vi "Material-Application-Dir-Metrics.vi"(11 "error in":errorcluster) -> (4 "Metrics Log Directory":path, 15 "error out":errorcluster)   [LabVIEW 2013]
uses:
  Material-Application-Dir-User.vi
panel:
  # "Inputs"
  # "Outputs"
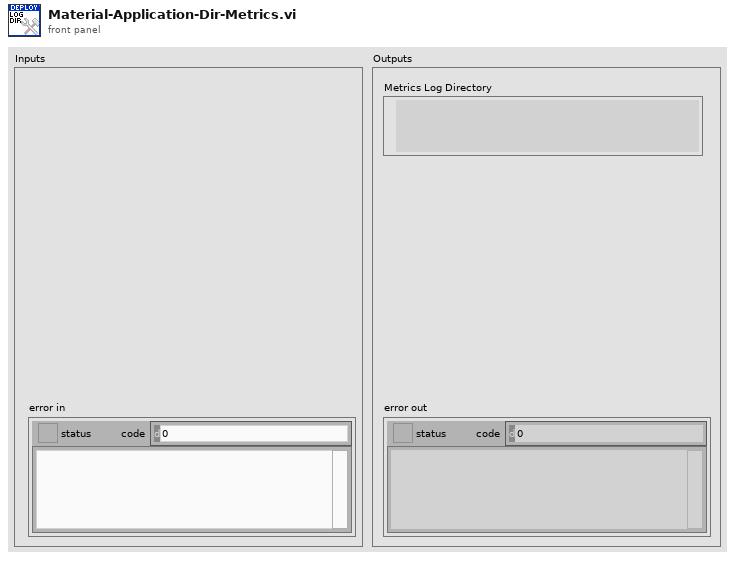
[diagram p1: front panel]
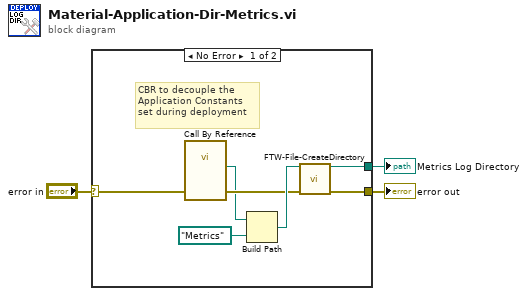
[diagram p0: block diagram]
diagram:
  n1 = case shown="No Error" "error in" {
    selector: "error in" -> [w6 w11]
    tunnel: [w9 w11] -> w3
    tunnel: [w8 _] -> w1
    frame No Error {
      # "CBR to decouple the\nApplication Constants\nset during deployment"
      n2 = call-by-ref "?"("error in"=w6) -> ("Deploy User App Data Directory"=w4:path, "error out"=w5:errorcluster)  [unwired: 15 in, 2 out]
      n3 = Build Path(base path=w4, name or relative path=path "Metrics" ("Subfolder")) -> (appended path=w10:path)
      n4 = call "FTW-File-CreateDirectory.vi"("Directory to Create"=w10, "error in"=w5) -> ("Created Directory"=w8:path, "error out"=w9:errorcluster)  [unwired: 12 in]
    }
    frame Error {
    }
  }
  "error out" <- w3
  "Metrics Log Directory" <- w1
